vi "Do Action.vi"(0 "Abstract Model in":refnum<class "Abstract Model.lvclass">, 7 "request":string, 11 "error in (no error)":errorcluster) -> (4 "Abstract Model out":refnum<class "Abstract Model.lvclass">, 15 "error out":errorcluster)   [LabVIEW 2022 SP3, in "Abstrat Model.lvlib" / "Abstract Model.lvclass"]
uses:
  Abstract Model.lvclass
  Abstract Model.lvclass/Abstract Model.ctl
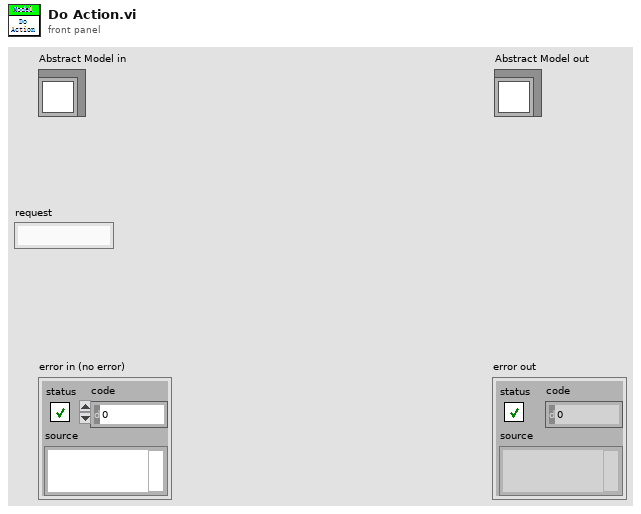
[diagram p1: front panel]
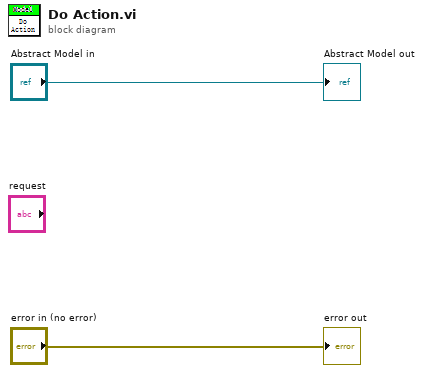
[diagram p0: block diagram]
diagram:
  "error out" <- "error in (no error)"
  "Abstract Model out" <- "Abstract Model in"
